vi "Chart View.vi"(10 "User Events in":refnum<class "User Events.lvclass">) -> ()   [LabVIEW 2015, in "FAMT Views.lvlib"]
uses:
  FAMT Views.lvlib
  User Events/User Events.lvclass
  User Events/User Events.lvclass/User Events.ctl
  Typedefs/State Types.ctl
  Typedefs/FAMT Typedefs.lvlib
panel:
  in  "Tab Control":enum32{"Translation", "Moment", "Cylinder"}(tab)
  out "Chart":T1(graph)
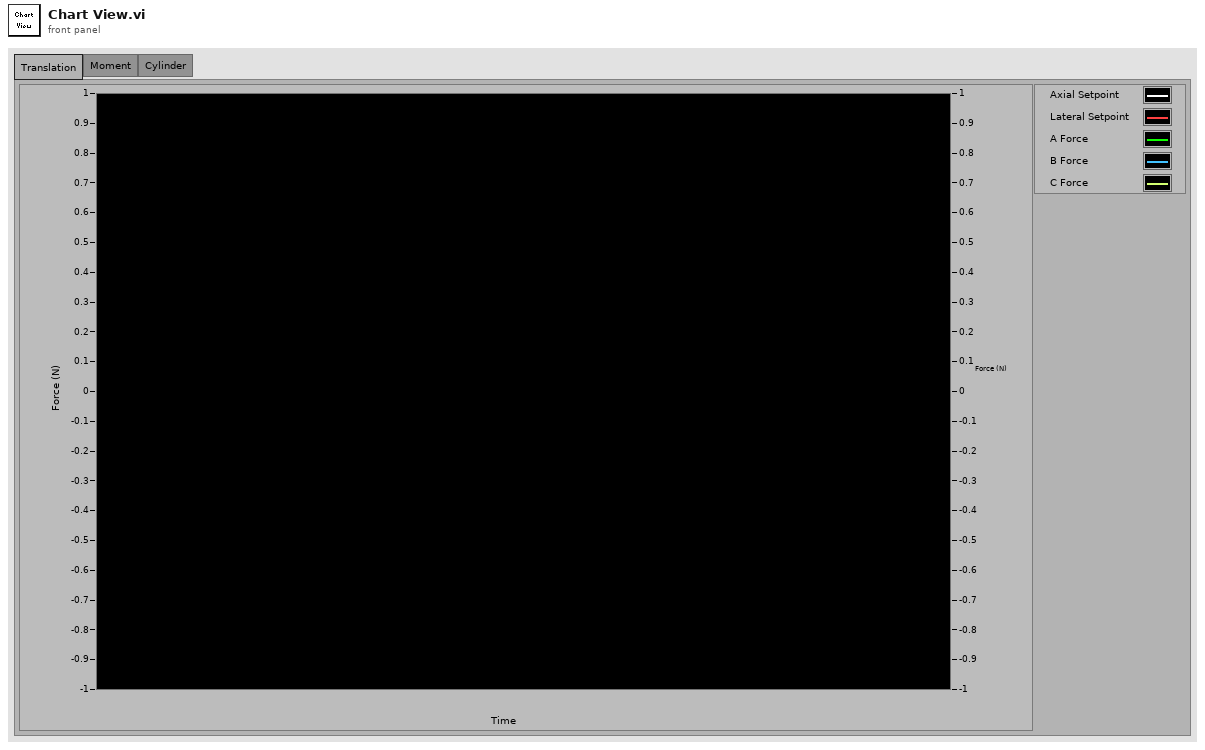
[diagram p1: front panel]
types:
  T1 = cluster{"Axial Demand":dbl, "Lateral Demand":dbl, dbl, dbl, dbl}
  T2 = typedef "FAMT Typedefs.lvlib/Publish Data Events.ctl" = cluster{"State":refnum<user-event>, "ErrorCode":refnum<user-event>, "FC1 ILC Outputs":refnum<user-event>, "LogPath":refnum<user-event>, "FC1 ILC Inputs":refnum<user-event>, "Scan Progress":refnum<user-event>, "FC2 ILC Outputs":refnum<user-event>, "FC2 ILC Inputs":refnum<user-event>}
  T3 = cluster{"Event Registration Refnum":refnum<event-registration>}
  T4 = typedef "FAMT Typedefs.lvlib/State Types.ctl" = enum16{"Offline State", "Fault State", "Standby State", "Disabled State", "Enabled State", "Wait For User Input State", "Perform Scan State"}
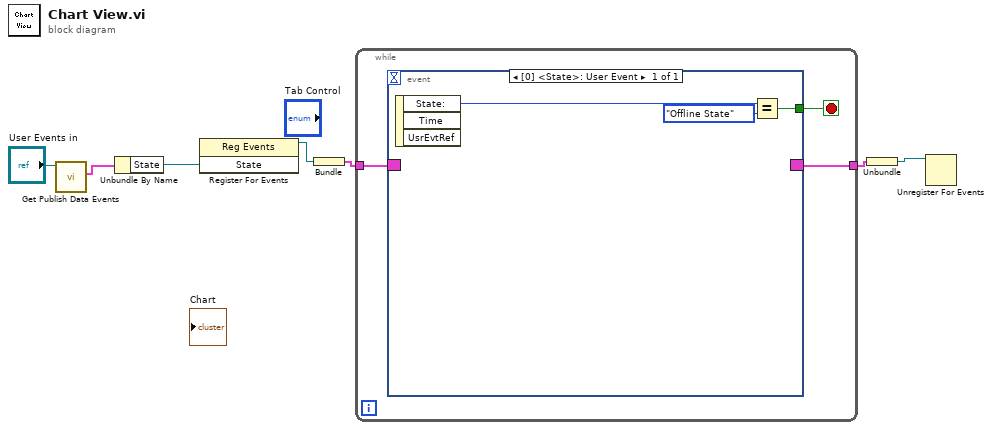
[diagram p0: block diagram]
diagram:
  n1 = call "Get Publish Data Events.vi"("UserEvents in"="User Events in") -> ("Publish Data Events"=w5:T2)  [unwired: 9 in, 1 out]
  n2 = Unbundle By Name(w5) -> ("State"=w6:refnum<user-event>)
  n3 = register-events(w6) -> (reference out=w7:refnum<event-registration>)  [unwired: 2 in, 1 out]
  n4 = Bundle("Event Registration Refnum"=w7) -> (w3:T3)  [unwired: 1 in]
  n5 = while {
    tunnel: w3 -> [w8]
    tunnel: [w10] -> w2
    stop <- w9 stop-if-true
    n6 = event shown="[0] <State>: User Event" {
      selector: w8 -> [_]
      dyn-events: [_] -> w10
      timeout: _ -> [_]
      tunnel: [w12] -> w9
      event User Event {
        n7 = event-data() -> ("State:"=w11:T4)  [unwired: 1 in, 2 out]
        n8 = Equal?(x=w11, y=State_Types."Offline State") -> (x = y?=w12:bool)
      }
    }
  }
  n9 = Unbundle(w2) -> ("Event Registration Refnum"=w4:refnum<event-registration>)
  n10 = Unregister For Events(event registration refnum=w4) -> ()  [unwired: 1 in, 1 out]
